vi "DataTransformM2C.vi"(2 "ERROR IN":errorcluster caption="错误输入（无错误）", 3 "MotorData":string) -> (0 "ERROR OUT":errorcluster caption="错误输出", 1 "Computer Data":dbl[](array[numeric]))   [LabVIEW 2016]
doc: "This is a data transforming VI, from motor data to computer data."
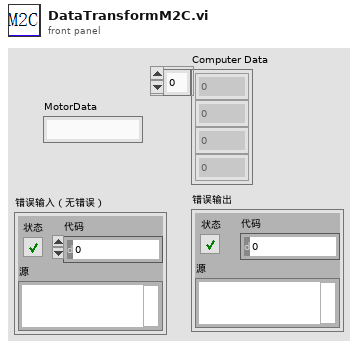
[diagram p1: front panel]
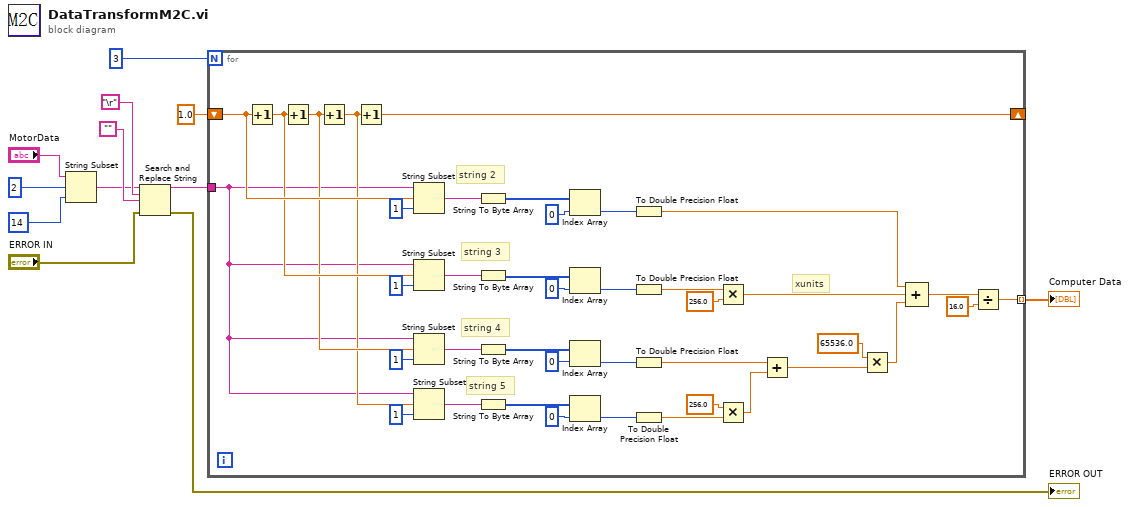
[diagram p0: block diagram]
diagram:
  n1 = String Subset(string="MotorData", offset (0)=2, length (rest)=14 ("length (rest)")) -> (substring=w5:string)
  n2 = Search and Replace String(input string=w5, search string="\r", replace string="", error in="ERROR IN") -> (result string=w3:string, error out=→"ERROR OUT":errorcluster)  [unwired: 4 in, 2 out]
  n3 = for {
    N: 3 -> [_]
    tunnel: [w19] -> w11 mode=indexing
    shift-right: [w14] -> _
    shift-left: 1.0 -> [w18]
    tunnel: w3 -> [w13]
    # "xunits"
    # "string 5"
    # "string 4"
    # "string 3"
    # "string 2"
    n4 = Increment(x=w18) -> (x+1=w17:dbl)
    n5 = Increment(x=w17) -> (x+1=w16:dbl)
    n6 = Increment(x=w16) -> (x+1=w15:dbl)
    n7 = Increment(x=w15) -> (x+1=w14:dbl)
    n8 = String Subset(string=w13, offset (0)=w18, length (rest)=1 ("length (rest)")) -> (substring=w51:string)
    n9 = String Subset(string=w13, offset (0)=w17, length (rest)=1 ("length (rest)")) -> (substring=w47:string)
    n10 = String Subset(string=w13, offset (0)=w16, length (rest)=1 ("length (rest)")) -> (substring=w43:string)
    n11 = String Subset(string=w13, offset (0)=w15, length (rest)=1 ("length (rest)")) -> (substring=w39:string)
    n12 = String To Byte Array(string=w51) -> (unsigned byte array=w50:u8[])
    n13 = String To Byte Array(string=w47) -> (unsigned byte array=w46:u8[])
    n14 = String To Byte Array(string=w43) -> (unsigned byte array=w42:u8[])
    n15 = String To Byte Array(string=w39) -> (unsigned byte array=w38:u8[])
    n16 = Index Array(array=w50, index=0) -> (element=w25:u8)
    n17 = Index Array(array=w46, index=0) -> (element=w28:u8)
    n18 = Index Array(array=w42, index=0) -> (element=w30:u8)
    n19 = Index Array(array=w38, index=0) -> (element=w34:u8)
    n20 = To Double Precision Float(number=w25) -> (double precision float=w24:dbl)
    n21 = To Double Precision Float(number=w28) -> (double precision float=w27:dbl)
    n22 = To Double Precision Float(number=w30) -> (double precision float=w31:dbl)
    n23 = To Double Precision Float(number=w34) -> (double precision float=w33:dbl)
    n24 = Multiply(x=w27, y=256.0) -> (x*y=w23:dbl)
    n25 = Multiply(x=256.0, y=w33) -> (x*y=w36:dbl)
    n26 = Add(x=w31, y=w36) -> (x+y=w35:dbl)
    n27 = Multiply(x=65536.0, y=w35) -> (x*y=w22:dbl)
    n28 = Compound Arithmetic op=ADD(w24, w23, w22) -> (w21:dbl)
    n29 = Divide(x=w21, y=16.0 ("x")) -> (x/y=w19:dbl)
  }
  "Computer Data" <- w11
